vi "Validate Variable Header.vi"(8 "error in (no error)":errorcluster, 11 "PUBLISH in":refnum<class "PUBLISH.lvclass">) -> (0 "error out":errorcluster, 1 "valid?":bool, 3 "PUBLISH out":refnum<class "PUBLISH.lvclass">)   [LabVIEW 2013, in "PUBLISH.lvclass"]
uses:
  PUBLISH.lvclass
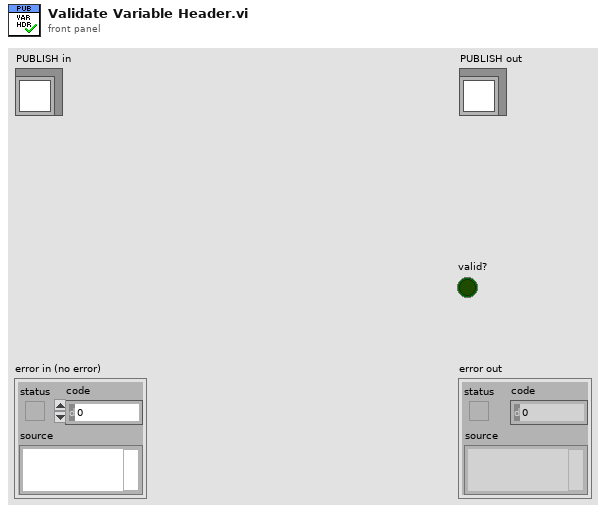
[diagram p1: front panel]
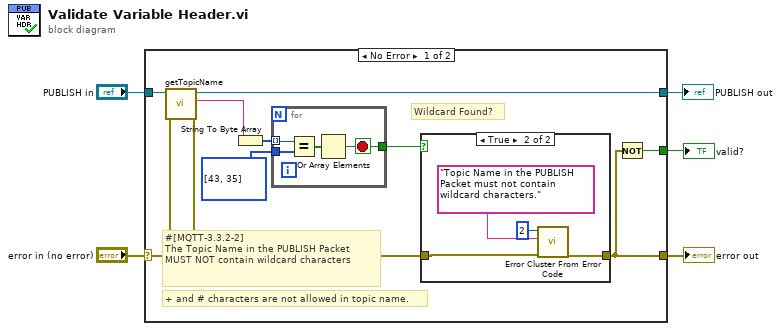
[diagram p0: block diagram]
diagram:
  n1 = case shown="No Error" "error in (no error)" {
    selector: "error in (no error)" -> [w13 w25]
    tunnel: "PUBLISH in" -> [w15 w26]
    tunnel: [w14 w26] -> w3
    tunnel: [w6 w25] -> w2
    tunnel: [w9 _] -> w1
    frame No Error {
      # "Wildcard Found?"
      # "+ and # characters are not allowed in topic name."
      # "#[MQTT-3.3.2-2]\nThe Topic Name in the PUBLISH Packet MUST NOT contain wildcard characters"
      n2 = call "getTopicName.vi"("error in (no error)"=w13, "PUBLISH in"=w15) -> ("error out"=w7:errorcluster, "Topic"=w12:string, "PUBLISH out"=w14:refnum<class "PUBLISH.lvclass">)  [unwired: 7 in]
      n3 = String To Byte Array(string=w12) -> (unsigned byte array=w11:u8[])
      n4 = for {
        tunnel: w11 -> [w24] mode=indexing
        tunnel: u8[] [43, 35] ("unsigned byte array") -> [w23]
        tunnel: [w21] -> w8
        stop <- w21 stop-if-true
        n5 = Equal?(x=w24, y=w23) -> (x = y?=w22:bool[])
        n6 = Or Array Elements(Boolean array=w22) -> (logical OR=w21:bool)
      }
      n7 = case shown="True" w8 {
        tunnel: w7 -> [w16 w19]
        tunnel: [w16 w20] -> w6
        frame False {
        }
        frame True {
          n8 = call <vilib>:"Error Cluster From Error Code.vi"("error in (no error)"=w19, "error message (\"\")"="Topic Name in the PUBLISH Packet must not contain wildcard characters.", "error code (0)"=2) -> ("error out"=w20:errorcluster)  [unwired: 6 in]
        }
      }
      n9 = Not(x=w6) -> (.not. x?=w9:bool)
    }
    frame Error {
    }
  }
  "error out" <- w2
  "PUBLISH out" <- w3
  "valid?" <- w1
